vi "例3_回原点运动.vi"() -> ()   [LabVIEW 2012]
panel:
  out "回零状态":string
  in  "软件复位":bool
  in  "硬件复位":bool
  out "负限位":bool
  out "正限位":bool
  out "原点":bool
  in  "回零偏移":dbl
  in  "总线状态":string
  in  "轴状态机":string
  in  "回零模式":dbl
  in  "退出程序":bool
  in  "卡号":dbl
  in  "位置清零":bool
  in  "立即停止":bool
  in  "减速停止":bool
  in  "启动":bool
  out "运动状态":string
  in  "当前位置 unit":dbl
  in  "当前速度 unit/s":dbl
  in  "减速时间 s":dbl
  in  "加速时间 s":dbl
  in  "回零高速 unit/s":dbl
  in  "回零低速 unit/s":dbl
  in  "电机轴号":dbl
  # "输入参数"
  # "信息显示"
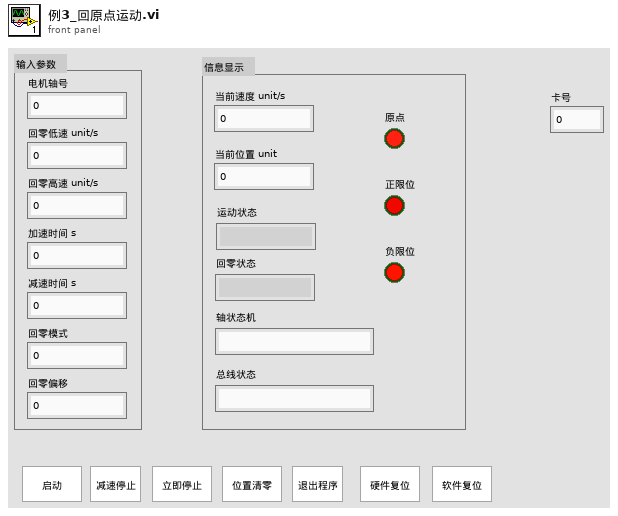
[diagram p1: front panel]
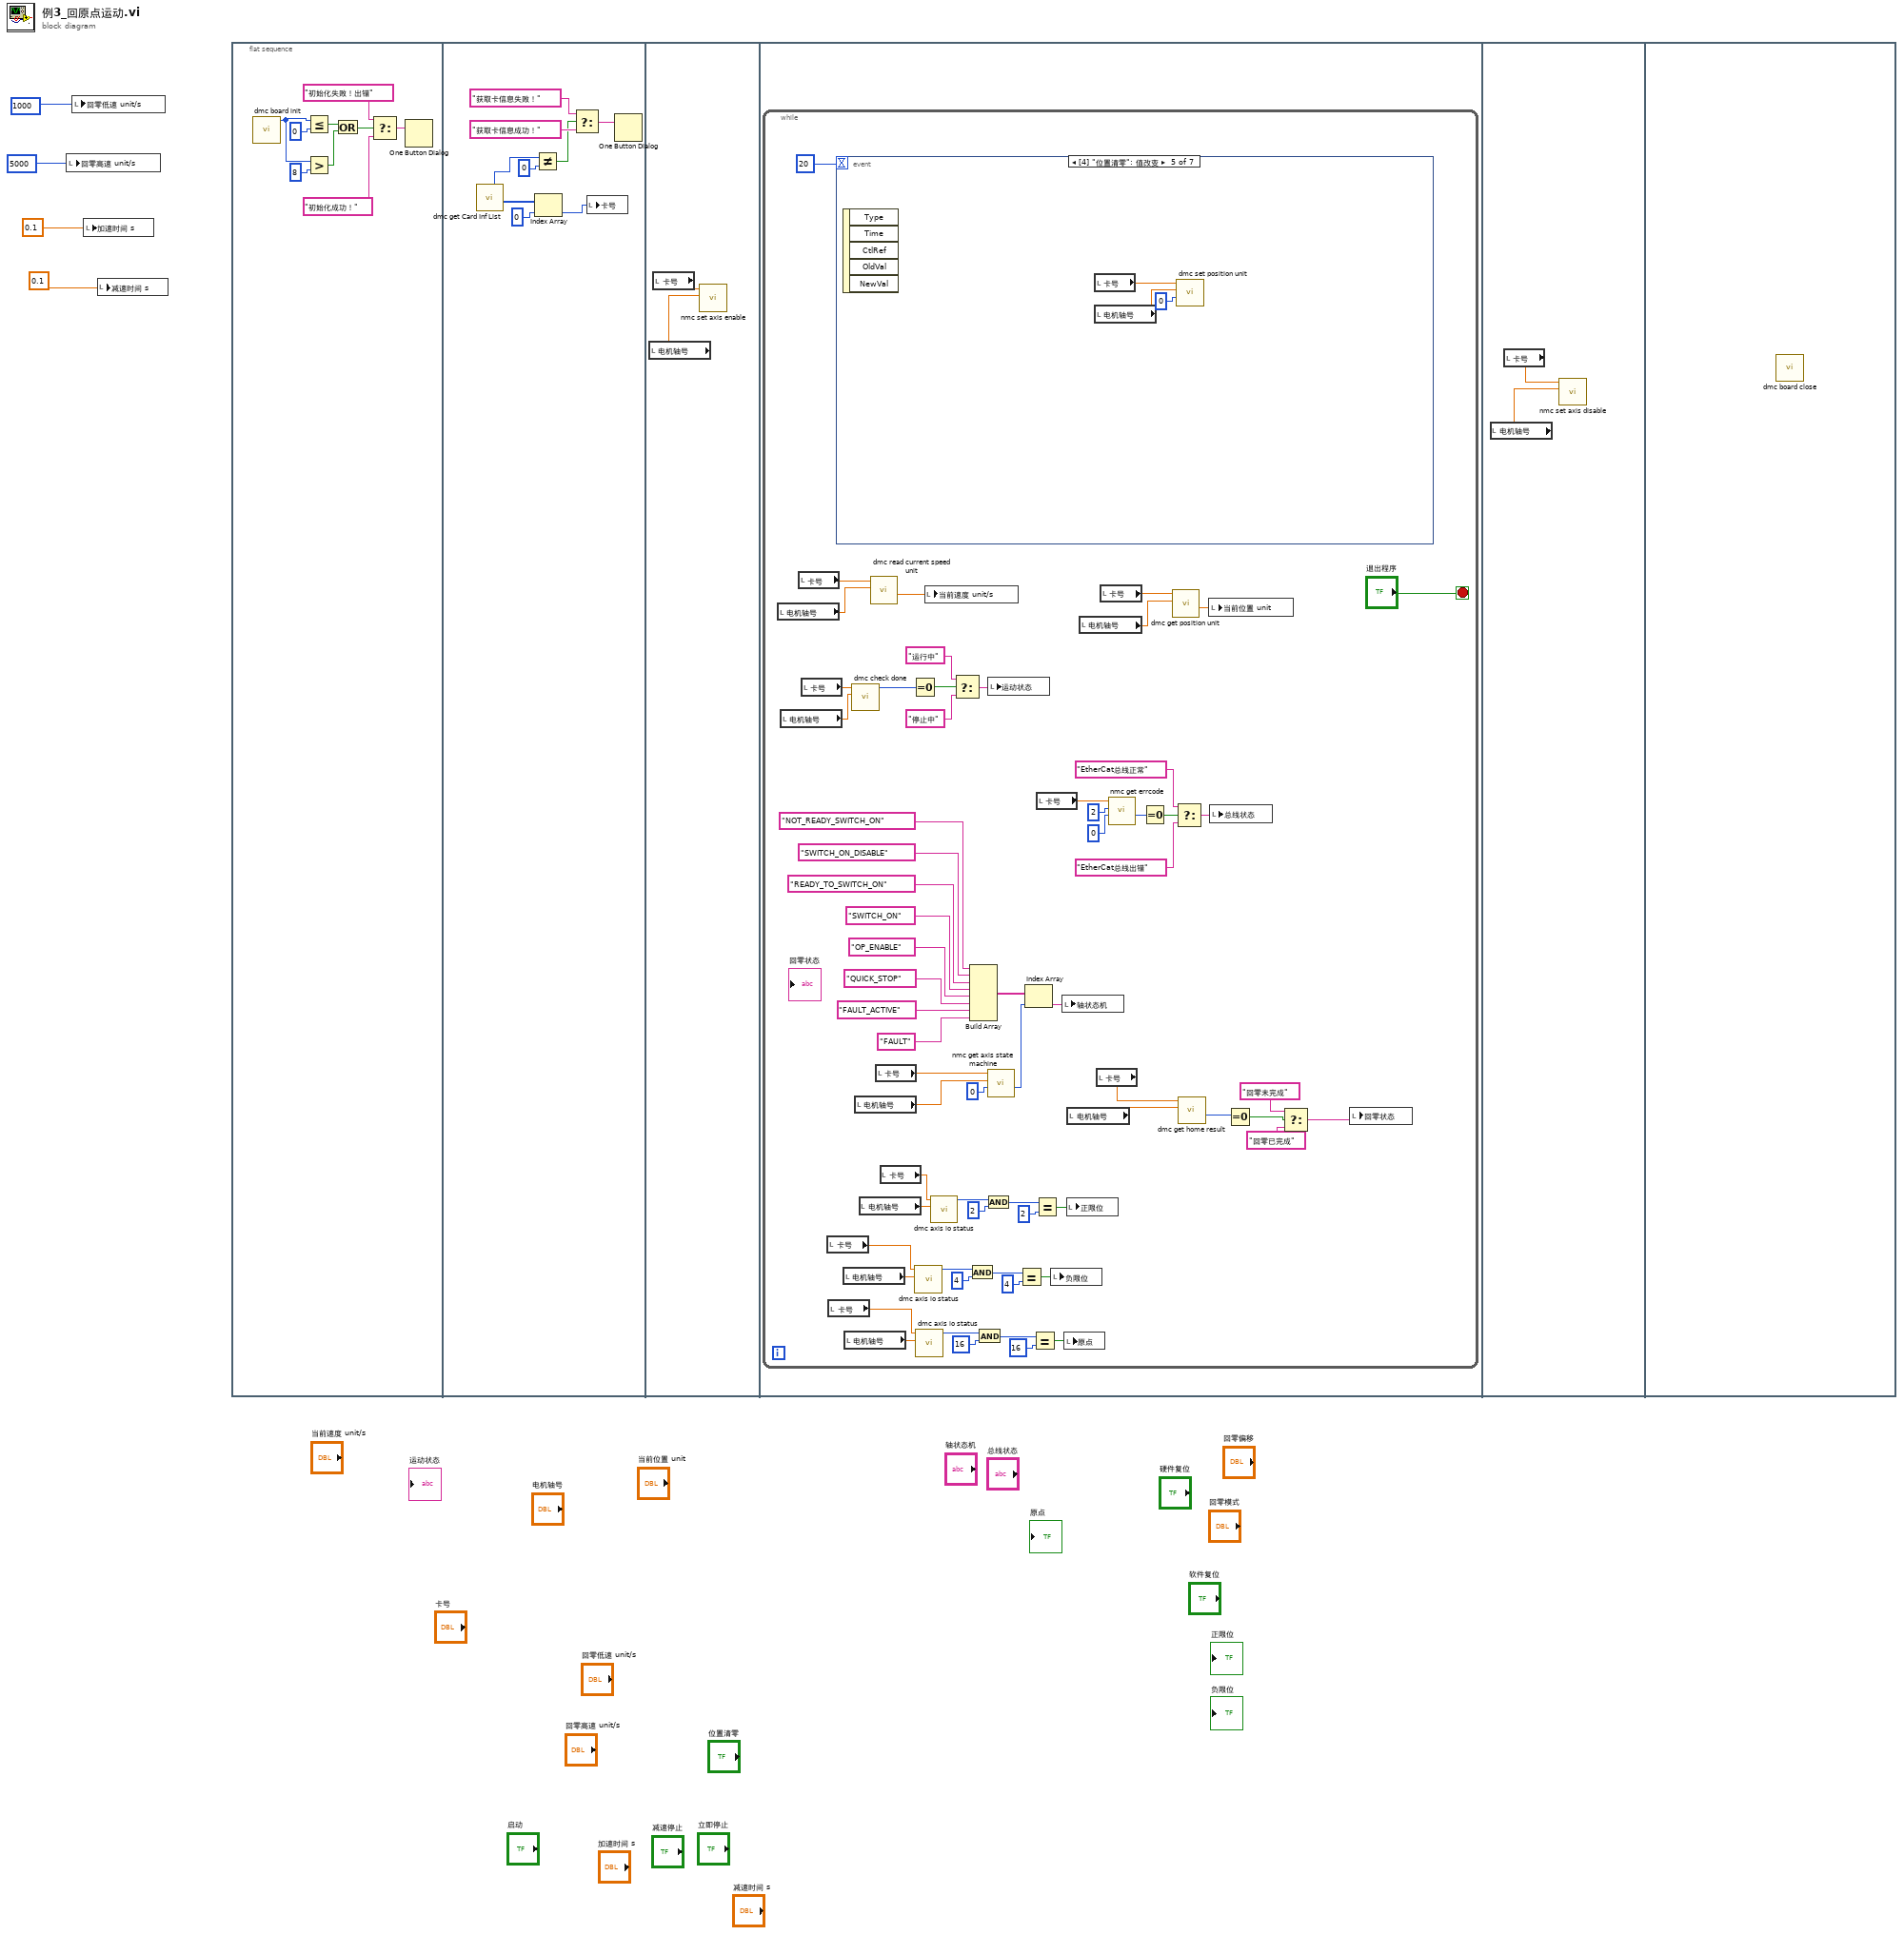
[diagram p0: block diagram]
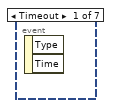
[diagram p2: hidden frame]
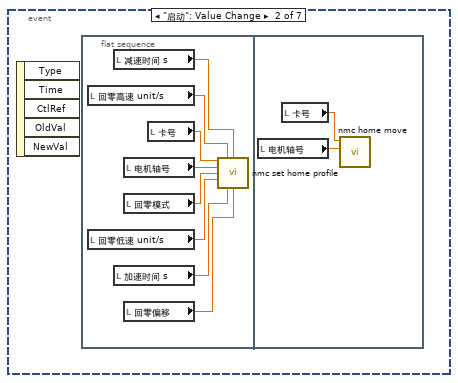
[diagram p3: hidden frame]
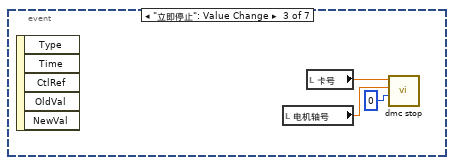
[diagram p4: hidden frame]
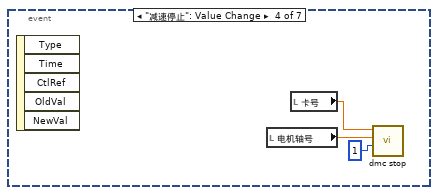
[diagram p5: hidden frame]
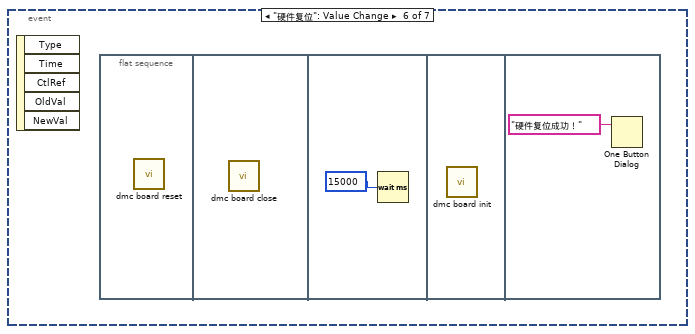
[diagram p6: hidden frame]
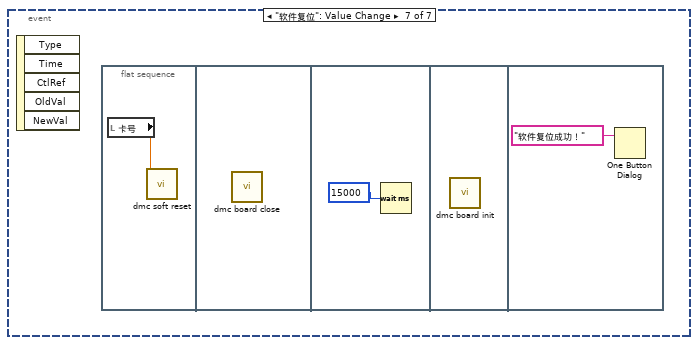
[diagram p7: hidden frame]
diagram:
  n1 = local write "回零高速 unit/s"(5000) -> ()
  n2 = local write "回零低速 unit/s"(1000) -> ()
  n3 = local write "加速时间 s"(0.1) -> ()
  n4 = local write "减速时间 s"(0.1) -> ()
  n5 = flat-sequence {
    frame #0 {
      n6 = call "dmc board init.vi"() -> ("function return"=w6:i16)  [unwired: 10 in, 1 out]
      n7 = Less Or Equal?(x=w6, y=0) -> (x <= y?=w9:bool)
      n8 = Greater?(x=w6, y=8) -> (0:w8:bool)
      n9 = Or(x=w9, y=w8) -> (x .or. y?=w10:bool)
      n10 = Select(t="初始化失败！出错", s=w10, f="初始化成功！") -> (s? t:f=w12:string)
      n11 = One Button Dialog(message=w12) -> ()  [unwired: 1 in, 1 out]
    }
    frame #1 {
      n12 = call "dmc get Card Inf List.vi"() -> ("CardIdList out"=w16:u16[], "function return"=w17:i16)  [unwired: 7 in, 3 out]
      n13 = Not Equal?(x=w17, y=0) -> (x != y?=w19:bool)
      n14 = Index Array(array=w16, index=0) -> (element=w14:u16)
      n15 = Select(t="获取卡信息失败！", s=w19, f="获取卡信息成功！") -> (s? t:f=w22:string)
      n16 = local write "卡号"(w14) -> ()
      n17 = One Button Dialog(message=w22) -> ()  [unwired: 1 in, 1 out]
    }
    frame #2 {
      n18 = local read "电机轴号"() -> (w23:dbl)
      n19 = local read "卡号"() -> (w24:dbl)
      n20 = call "nmc set axis enable.vi"("axis"=w23, "CardNo"=w24) -> ()  [unwired: 8 in, 2 out]
    }
    frame #3 {
      n21 = while {
        stop <- "退出程序" stop-if-true
        n22 = local read "电机轴号"() -> (w83:dbl)
        n23 = local read "电机轴号"() -> (w79:dbl)
        n24 = local read "卡号"() -> (w84:dbl)
        n25 = local read "卡号"() -> (w80:dbl)
        n26 = local read "卡号"() -> (w39:dbl)
        n27 = local read "卡号"() -> (w36:dbl)
        n28 = event shown="[4] \"位置清零\": 值改变" {
          selector: _ -> [_ _ _ _ _ _ _]
          dyn-events: _ -> [_ _ _ _ _ _ _]
          timeout: 20 -> [_ _ _ _ _ _ _]
          event Timeout {
            n29 = event-data() -> ()  [unwired: 1 in, 2 out]
          }
          event "启动": Value Change {
            n30 = event-data() -> ()  [unwired: 1 in, 5 out]
            n31 = flat-sequence {
              frame #0 {
                n32 = local read "回零高速 unit/s"() -> (w93:dbl)
                n33 = local read "回零低速 unit/s"() -> (w94:dbl)
                n34 = local read "减速时间 s"() -> (w92:dbl)
                n35 = local read "加速时间 s"() -> (w91:dbl)
                n36 = local read "电机轴号"() -> (w96:dbl)
                n37 = local read "回零模式"() -> (w95:dbl)
                n38 = local read "回零偏移"() -> (w90:dbl)
                n39 = local read "卡号"() -> (w97:dbl)
                n40 = call "nmc set home profile.vi"("CardNo"=w97, "High_Vel"=w93, "Tdec"=w92, "axis"=w96, "home_mode"=w95, "Low_Vel"=w94, "Tacc"=w91, "offsetpos"=w90) -> ()  [unwired: 6 in, 2 out]
              }
              frame #1 {
                n41 = local read "电机轴号"() -> (w98:dbl)
                n42 = local read "卡号"() -> (w99:dbl)
                n43 = call "nmc home move.vi"("axis"=w98, "CardNo"=w99) -> ()  [unwired: 8 in, 2 out]
              }
            }
          }
          event "立即停止": Value Change {
            n44 = event-data() -> ()  [unwired: 1 in, 5 out]
            n45 = local read "电机轴号"() -> (w101:dbl)
            n46 = local read "卡号"() -> (w100:dbl)
            n47 = call "dmc stop.vi"("stop_mode"=0, "axis"=w101, "CardNo"=w100) -> ()  [unwired: 7 in, 2 out]
          }
          event "减速停止": Value Change {
            n48 = event-data() -> ()  [unwired: 1 in, 5 out]
            n49 = local read "电机轴号"() -> (w104:dbl)
            n50 = local read "卡号"() -> (w103:dbl)
            n51 = call "dmc stop.vi"("stop_mode"=1, "axis"=w104, "CardNo"=w103) -> ()  [unwired: 7 in, 2 out]
          }
          event "位置清零": Value Change {
            n52 = event-data() -> ()  [unwired: 1 in, 5 out]
            n53 = local read "卡号"() -> (w106:dbl)
            n54 = local read "电机轴号"() -> (w107:dbl)
            n55 = call "dmc set position unit.vi"("pos"=0, "axis"=w107, "CardNo"=w106) -> ()  [unwired: 7 in, 2 out]
          }
          event "硬件复位": Value Change {
            n56 = event-data() -> ()  [unwired: 1 in, 5 out]
            n57 = flat-sequence {
              frame #0 {
                n58 = call "dmc board reset.vi"() -> ()  [unwired: 10 in, 2 out]
              }
              frame #1 {
                n59 = call "dmc board close.vi"() -> ()  [unwired: 10 in, 2 out]
              }
              frame #2 {
                n60 = Wait (ms)(milliseconds to wait=15000) -> ()  [unwired: 1 out]
              }
              frame #3 {
                n61 = call "dmc board init.vi"() -> ()  [unwired: 10 in, 2 out]
              }
              frame #4 {
                n62 = One Button Dialog(message="硬件复位成功！") -> ()  [unwired: 1 in, 1 out]
              }
            }
          }
          event "软件复位": Value Change {
            n63 = event-data() -> ()  [unwired: 1 in, 5 out]
            n64 = flat-sequence {
              frame #0 {
                n65 = local read "卡号"() -> (w111:dbl)
                n66 = call "dmc soft reset.vi"("CardNo"=w111) -> ()  [unwired: 9 in, 2 out]
              }
              frame #1 {
                n67 = call "dmc board close.vi"() -> ()  [unwired: 10 in, 2 out]
              }
              frame #2 {
                n68 = Wait (ms)(milliseconds to wait=15000) -> ()  [unwired: 1 out]
              }
              frame #3 {
                n69 = call "dmc board init.vi"() -> ()  [unwired: 10 in, 2 out]
              }
              frame #4 {
                n70 = One Button Dialog(message="软件复位成功！") -> ()  [unwired: 1 in, 1 out]
              }
            }
          }
        }
        n71 = local read "电机轴号"() -> (w38:dbl)
        n72 = local read "电机轴号"() -> (w37:dbl)
        n73 = call "dmc check done.vi"("axis"=w79, "CardNo"=w80) -> ("function return"=w85:i16)  [unwired: 8 in, 1 out]
        n74 = local read "电机轴号"() -> (w64:dbl)
        n75 = local read "电机轴号"() -> (w54:dbl)
        n76 = call "dmc read current speed unit.vi"("axis"=w83, "CardNo"=w84) -> ("current_speed out"=w26:dbl)  [unwired: 7 in, 2 out]
        n77 = local read "卡号"() -> (w65:dbl)
        n78 = local read "卡号"() -> (w53:dbl)
        n79 = Equal To 0?(x=w85) -> (x = 0?=w88:bool)
        n80 = call "dmc axis io status.vi"("axis"=w38, "CardNo"=w39) -> ("function return"=w47:u32)  [unwired: 8 in, 1 out]
        n81 = call "dmc axis io status.vi"("axis"=w37, "CardNo"=w36) -> ("function return"=w43:u32)  [unwired: 8 in, 1 out]
        n82 = local write "当前速度 unit/s"(w26) -> ()
        n83 = call "dmc axis io status.vi"("axis"=w54, "CardNo"=w53) -> ("function return"=w52:u32)  [unwired: 8 in, 1 out]
        n84 = Select(t="运行中" ("当前状态"), s=w88, f="停止中" ("当前状态")) -> (s? t:f=w78:string)
        n85 = And(x=w47, y=4) -> (x .and. y?=w45:u32)
        n86 = Build Array("NOT_READY_SWITCH_ON", "SWITCH_ON_DISABLE", "READY_TO_SWITCH_ON", "SWITCH_ON", "OP_ENABLE", "QUICK_STOP", "FAULT_ACTIVE", "FAULT") -> (w68:string[])
        n87 = And(x=w43, y=16) -> (x .and. y?=w41:u32)
        n88 = And(x=w52, y=2) -> (x .and. y?=w50:u32)
        n89 = local write "运动状态"(w78) -> ()
        n90 = call "nmc get axis state machine.vi"("Axis_StateMachine"=0, "axis"=w64, "CardNo"=w65) -> ("Axis_StateMachine out"=w67:u16)  [unwired: 6 in, 2 out]
        n91 = Equal?(x=w45, y=4) -> (x = y?=w35:bool)
        n92 = Index Array(array=w68, index=w67) -> (element=w63:string)
        n93 = Equal?(x=w41, y=16) -> (x = y?=w34:bool)
        n94 = Equal?(x=w50, y=2) -> (x = y?=w48:bool)
        n95 = local read "卡号"() -> (w56:dbl)
        n96 = local write "负限位"(w35) -> ()
        n97 = local write "轴状态机"(w63) -> ()
        n98 = local write "原点"(w34) -> ()
        n99 = local write "正限位"(w48) -> ()
        n100 = local read "电机轴号"() -> (w32:dbl)
        n101 = local read "电机轴号"() -> (w82:dbl)
        n102 = local read "卡号"() -> (w33:dbl)
        n103 = local read "卡号"() -> (w81:dbl)
        n104 = call "nmc get errcode.vi"("Errcode"=0, "channel"=2, "CardNo"=w56) -> ("Errcode out"=w62:u16)  [unwired: 6 in, 2 out]
        n105 = Equal To 0?(x=w62) -> (x = 0?=w61:bool)
        n106 = call "dmc get position unit.vi"("axis"=w82, "CardNo"=w81) -> ("pos out"=w25:dbl)  [unwired: 7 in, 2 out]
        n107 = Select(t="EtherCat总线正常" ("当前状态"), s=w61, f="EtherCat总线出错" ("当前状态")) -> (s? t:f=w55:string)
        n108 = call "dmc get home result.vi"("axis"=w32, "CardNo"=w33) -> ("state out"=w31:u16)  [unwired: 7 in, 2 out]
        n109 = local write "当前位置 unit"(w25) -> ()
        n110 = local write "总线状态"(w55) -> ()
        n111 = Equal To 0?(x=w31) -> (x = 0?=w30:bool)
        n112 = Select(t="回零未完成" ("当前状态"), s=w30, f="回零已完成" ("当前状态")) -> (s? t:f=w27:string)
        n113 = local write "回零状态"(w27) -> ()
      }
    }
    frame #4 {
      n114 = local read "电机轴号"() -> (w114:dbl)
      n115 = local read "卡号"() -> (w115:dbl)
      n116 = call "nmc set axis disable.vi"("axis"=w114, "CardNo"=w115) -> ()  [unwired: 8 in, 2 out]
    }
    frame #5 {
      n117 = call "dmc board close.vi"() -> ()  [unwired: 10 in, 2 out]
    }
  }
